vi "test1.vi"() -> ()   [LabVIEW 2016]
panel:
  out "x+y":dbl
  out "ReturnValue":u32
  in  "Device Type":u16(ring) items=["PCI-1285 (M0)"]
  in  "Distance":dbl
  out "AxisHandle":u32
  out "DeviceNum List":u32[](array[numeric])
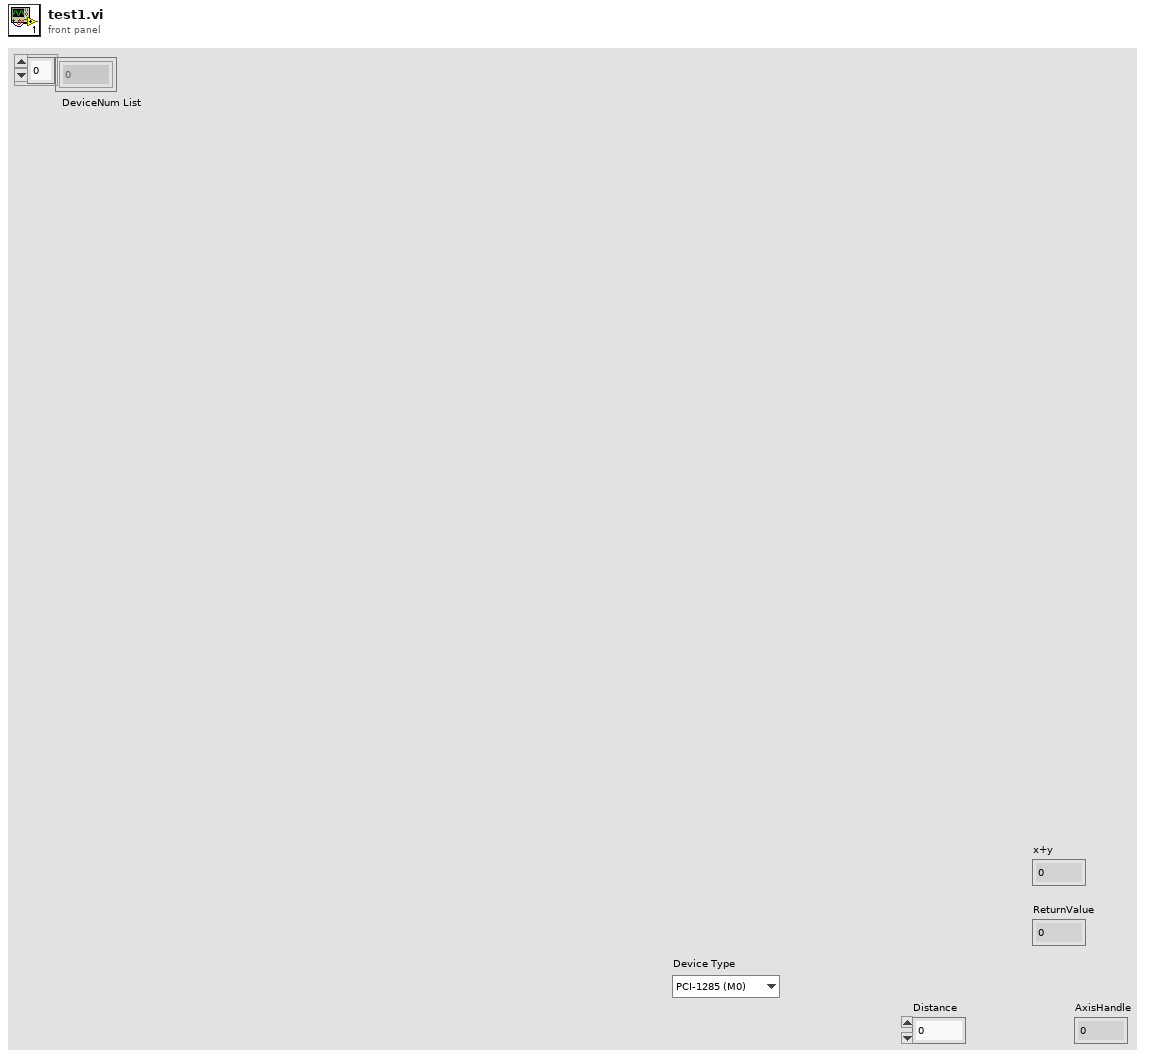
[diagram p1: front panel]
types:
  T1 = cluster{"DeviceNum":u32, "U*8 Array":cluster{"U*8 Array[0]":u8, "U*8 Array[1]":u8, "U*8 Array[2]":u8, "U*8 Array[3]":u8, "U*8 Array[4]":u8, "U*8 Array[5]":u8, "U*8 Array[6]":u8, "U*8 Array[7]":u8, "U*8 Array[8]":u8, "U*8 Array[9]":u8, "U*8 Array[10]":u8, "U*8 Array[11]":u8, "U*8 Array[12]":u8, "U*8 Array[13]":u8, "U*8 Array[14]":u8, "U*8 Array[15]":u8, "U*8 Array[16]":u8, "U*8 Array[17]":u8, "U*8 Array[18]":u8, "U*8 Array[19]":u8, "U*8 Array[20]":u8, "U*8 Array[21]":u8, "U*8 Array[22]":u8, "U*8 Array[23]":u8, "U*8 Array[24]":u8, "U*8 Array[25]":u8, "U*8 Array[26]":u8, "U*8 Array[27]":u8, "U*8 Array[28]":u8, "U*8 Array[29]":u8, "U*8 Array[30]":u8, "U*8 Array[31]":u8, "U*8 Array[32]":u8, "U*8 Array[33]":u8, "U*8 Array[34]":u8, "U*8 Array[35]":u8, "U*8 Array[36]":u8, "U*8 Array[37]":u8, "U*8 Array[38]":u8, "U*8 Array[39]":u8, "U*8 Array[40]":u8, "U*8 Array[41]":u8, "U*8 Array[42]":u8, "U*8 Array[43]":u8, "U*8 Array[44]":u8, "U*8 Array[45]":u8, "U*8 Array[46]":u8, "U*8 Array[47]":u8, "U*8 Array[48]":u8, "U*8 Array[49]":u8}, "NumOfSubDevice":i16}[]
  T2 = cluster{"U*8 Array[0]":u8, "U*8 Array[1]":u8, "U*8 Array[2]":u8, "U*8 Array[3]":u8, "U*8 Array[4]":u8, "U*8 Array[5]":u8, "U*8 Array[6]":u8, "U*8 Array[7]":u8, "U*8 Array[8]":u8, "U*8 Array[9]":u8, "U*8 Array[10]":u8, "U*8 Array[11]":u8, "U*8 Array[12]":u8, "U*8 Array[13]":u8, "U*8 Array[14]":u8, "U*8 Array[15]":u8, "U*8 Array[16]":u8, "U*8 Array[17]":u8, "U*8 Array[18]":u8, "U*8 Array[19]":u8, "U*8 Array[20]":u8, "U*8 Array[21]":u8, "U*8 Array[22]":u8, "U*8 Array[23]":u8, "U*8 Array[24]":u8, "U*8 Array[25]":u8, "U*8 Array[26]":u8, "U*8 Array[27]":u8, "U*8 Array[28]":u8, "U*8 Array[29]":u8, "U*8 Array[30]":u8, "U*8 Array[31]":u8, "U*8 Array[32]":u8, "U*8 Array[33]":u8, "U*8 Array[34]":u8, "U*8 Array[35]":u8, "U*8 Array[36]":u8, "U*8 Array[37]":u8, "U*8 Array[38]":u8, "U*8 Array[39]":u8, "U*8 Array[40]":u8, "U*8 Array[41]":u8, "U*8 Array[42]":u8, "U*8 Array[43]":u8, "U*8 Array[44]":u8, "U*8 Array[45]":u8, "U*8 Array[46]":u8, "U*8 Array[47]":u8, "U*8 Array[48]":u8, "U*8 Array[49]":u8}
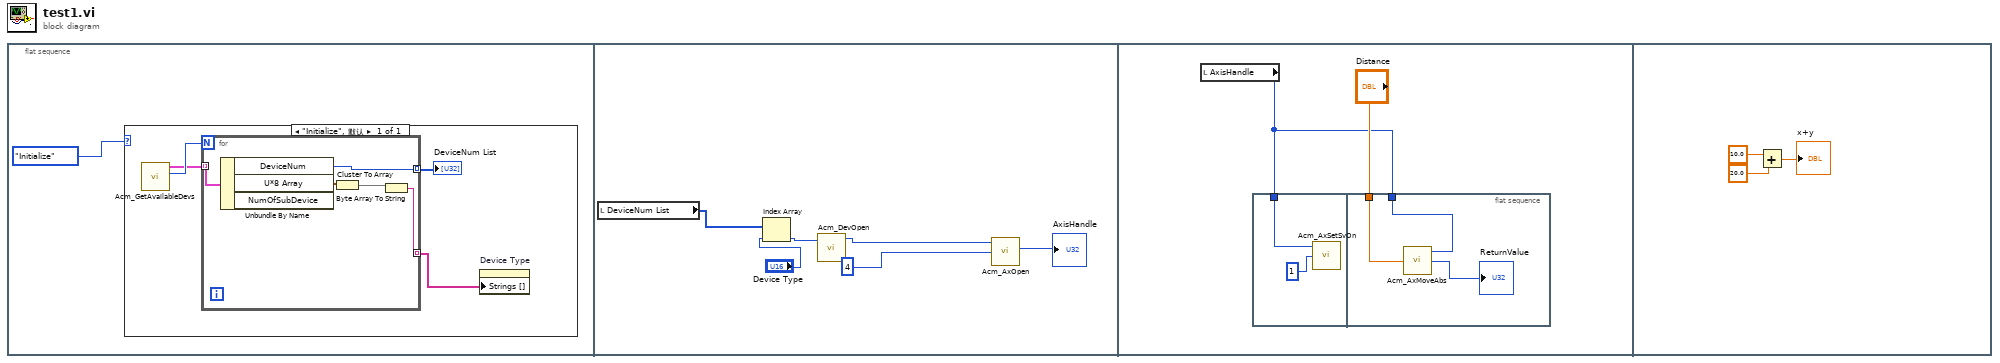
[diagram p0: block diagram]
diagram:
  n1 = flat-sequence {
    frame #0 {
      n2 = case shown="\"Initialize\", 默认" enum16{"Initialize"}."Initialize" ("Enum") {
        frame "Initialize", Default {
          n3 = call <userlib>:"Acm_GetAvailableDevs.vi"() -> ("DeviceList"=w4:T1, "OutEntries"=w5:u32)  [unwired: 1 in, 4 out]
          n4 = for {
            N: w5 -> [_]
            tunnel: w4 -> [w10] mode=indexing
            tunnel: [w7] -> w3 mode=indexing
            tunnel: [w6] -> w2 mode=indexing
            n5 = Unbundle By Name(w10) -> ("DeviceNum"=w7:u32, "U*8 Array"=w9:T2)  [unwired: 1 out]
            n6 = Cluster To Array(cluster=w9) -> (array=w8:u8[])
            n7 = Byte Array To String(unsigned byte array=w8) -> (string=w6:string)
          }
          "DeviceNum List" <- w3
          n8 = property on="Device Type" class="Ring (严格)"("Strings []"=w2) -> ()  [unwired: 2 in, 2 out]
        }
      }
    }
    frame #1 {
      n9 = local read "DeviceNum List"() -> (w12:u32[])
      n10 = Index Array(array=w12, index="Device Type") -> (element=w11:u32)
      n11 = call <userlib>:"Acm_DevOpen.vi"("DeviceNumber"=w11) -> ("DeviceHandle"=w13:u32)  [unwired: 1 in, 2 out]
      n12 = call <userlib>:"Acm_AxOpen.vi"("PhyAxis"=u16 4, "DeviceHandle"=w13) -> ("AxisHandle"=→"AxisHandle":u32)  [unwired: 1 in, 3 out]
    }
    frame #2 {
      n13 = local read "AxisHandle"() -> (w17:u32)
      n14 = flat-sequence {
        tunnel: w17 -> [w20]
        tunnel: w17 -> [w23]
        tunnel: "Distance" -> [w22]
        frame #0 {
          n15 = call <userlib>:"Acm_AxSetSvOn.vi"("OnOff"=u32 1, "AxisHandle"=w20) -> ()  [unwired: 1 in, 3 out]
        }
        frame #1 {
          n16 = call <userlib>:"Acm_AxMoveAbs.vi"("Position"=w22, "AxisHandle"=w23) -> ("ReturnValue"=→"ReturnValue":u32)  [unwired: 1 in, 2 out]
        }
      }
    }
    frame #3 {
      n17 = Add(x=10.0, y=20.0) -> (x+y=→"x+y":dbl)
    }
  }
